vi "wsReadAccessToken.vi"(8 "error in (no error)":errorcluster) -> (0 "error out":errorcluster, 2 "Found?":bool, 3 "access token":string)   [LabVIEW 2018, in "HASS-LV-WS_integration.lvlib"]
uses:
  HASS-LV-WS_integration.lvlib
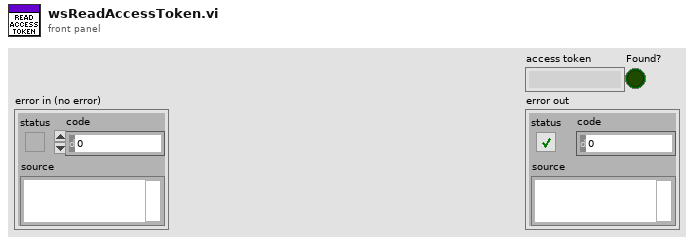
[diagram p1: front panel]
types:
  T1 = enum16{"open", "replace", "create", "open or create", "replace or create", "replace or create with confirmation"}
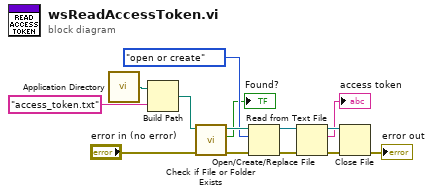
[diagram p0: block diagram]
diagram:
  n1 = call <vilib>:"Application Directory.vi"() -> ("Application Directory"=w14:path)
  n2 = Build Path(base path=w14, name or relative path="access_token.txt") -> (appended path=w13:path)
  n3 = call <vilib>:"Check if File or Folder Exists.vi"("error in (no error)"="error in (no error)", "path"=w13) -> ("error out"=w10:errorcluster, "file or folder exists?"=→"Found?":bool, "dup path"=w11:path)  [unwired: 7 in]
  n4 = Open/Create/Replace File(file path (use dialog)=w11, error in=w10, operation (0:open)=T1."open or create") -> (refnum out=w8:refnum<file>, error out=w9:errorcluster)  [unwired: 3 in, 1 out]
  n5 = Read from Text File(file (use dialog)=w8, error in=w9) -> (refnum out=w6:refnum<file>, text=→"access token":string, error out=w7:errorcluster)  [unwired: 2 in, 1 out]
  n6 = Close File(refnum=w6, error in=w7) -> (error out=→"error out":errorcluster)  [unwired: 1 out]
